vi "DeleteFF.vi"(9 "Count":i32, 10 "Data":u8[](array[numeric]) format="%.0x") -> (2 "Data out":u8[](array[numeric]) format="%.0x")   [LabVIEW 2018]
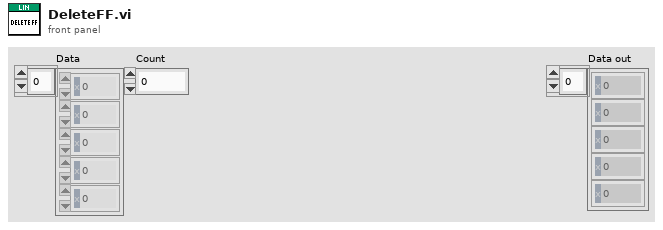
[diagram p1: front panel]
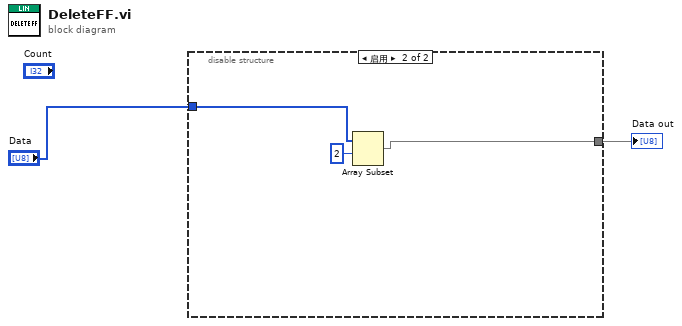
[diagram p0: block diagram]
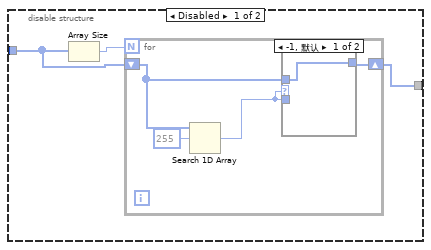
[diagram p2: hidden frame]
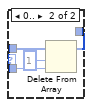
[diagram p3: hidden frame]
diagram:
  n1 = disable-structure shown="启用" {
    disable-tunnel: [w5 w15] -> w2
    disable-tunnel: "Data" -> [w4 w17]
    frame Disabled {
      n2 = Array Size(array=w4) -> (size(s)=w3:i32)
      n3 = for {
        N: w3 -> [_]
        shift-right: [w7] -> w5
        shift-left: w4 -> [w8]
        n4 = Search 1D Array(1D array=w8, element=u8 255 ("元素")) -> (index of element=w6:i32)  [unwired: 1 in]
        n5 = case shown="-1, 默认" w6 {
          tunnel: w8 -> [w10 w14]
          tunnel: w6 -> [_ w13]
          tunnel: [w10 w11] -> w7
          frame -1, Default {
          }
          frame 0.. {
            n6 = Delete From Array(array=w14, length=1 ("长度"), index=w13) -> (array with subset deleted=w11:u8[])  [unwired: 1 out]
          }
        }
      }
    }
    frame Enabled {
      n7 = Array Subset(array=w17, index=2 ("索引")) -> (w15:u8[])  [unwired: 1 in]
    }
  }
  "Data out" <- w2
